vi "Delay Line.vi"() -> ()   [LabVIEW 2013]
uses:
  PI Globals/MercuryConfigured.vi
  PI Globals/ControllerIdentification.vi
  PI Globals/MovementRange.vi
  PI Globals/ConnectedAxes.vi
panel:
  in  "Clear Error":bool
  out "Current velocity":dbl
  in  "Set Velocity":bool
  in  "Set Vel.":dbl
  in  "Query Velocity":bool
  in  "Start":bool
  out "Ready?":bool=TRUE
  in  "JOG +":bool
  out "Conn. \nAxes":string[](array[string])
  in  "Go":bool
  in  "Position to reach":dbl
  in  "Step Size (mm)":dbl
  in  "JOG -":bool
  out "Serial Number":string
  out "Identification":string
  out "+/- Movement range":dbl
  out "error out":errorcluster
  in  "Query Pos.":bool
  out "Position de la ligne à retard":dbl(slide) min=-51.0 max=51.0 scale=0.0..100.0
  in  "error in":errorcluster
  in  "stop":bool
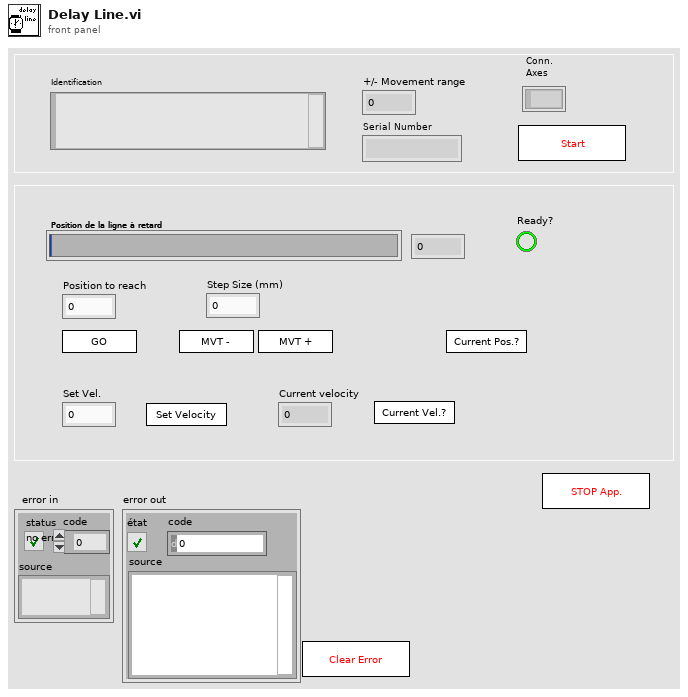
[diagram p1: front panel]
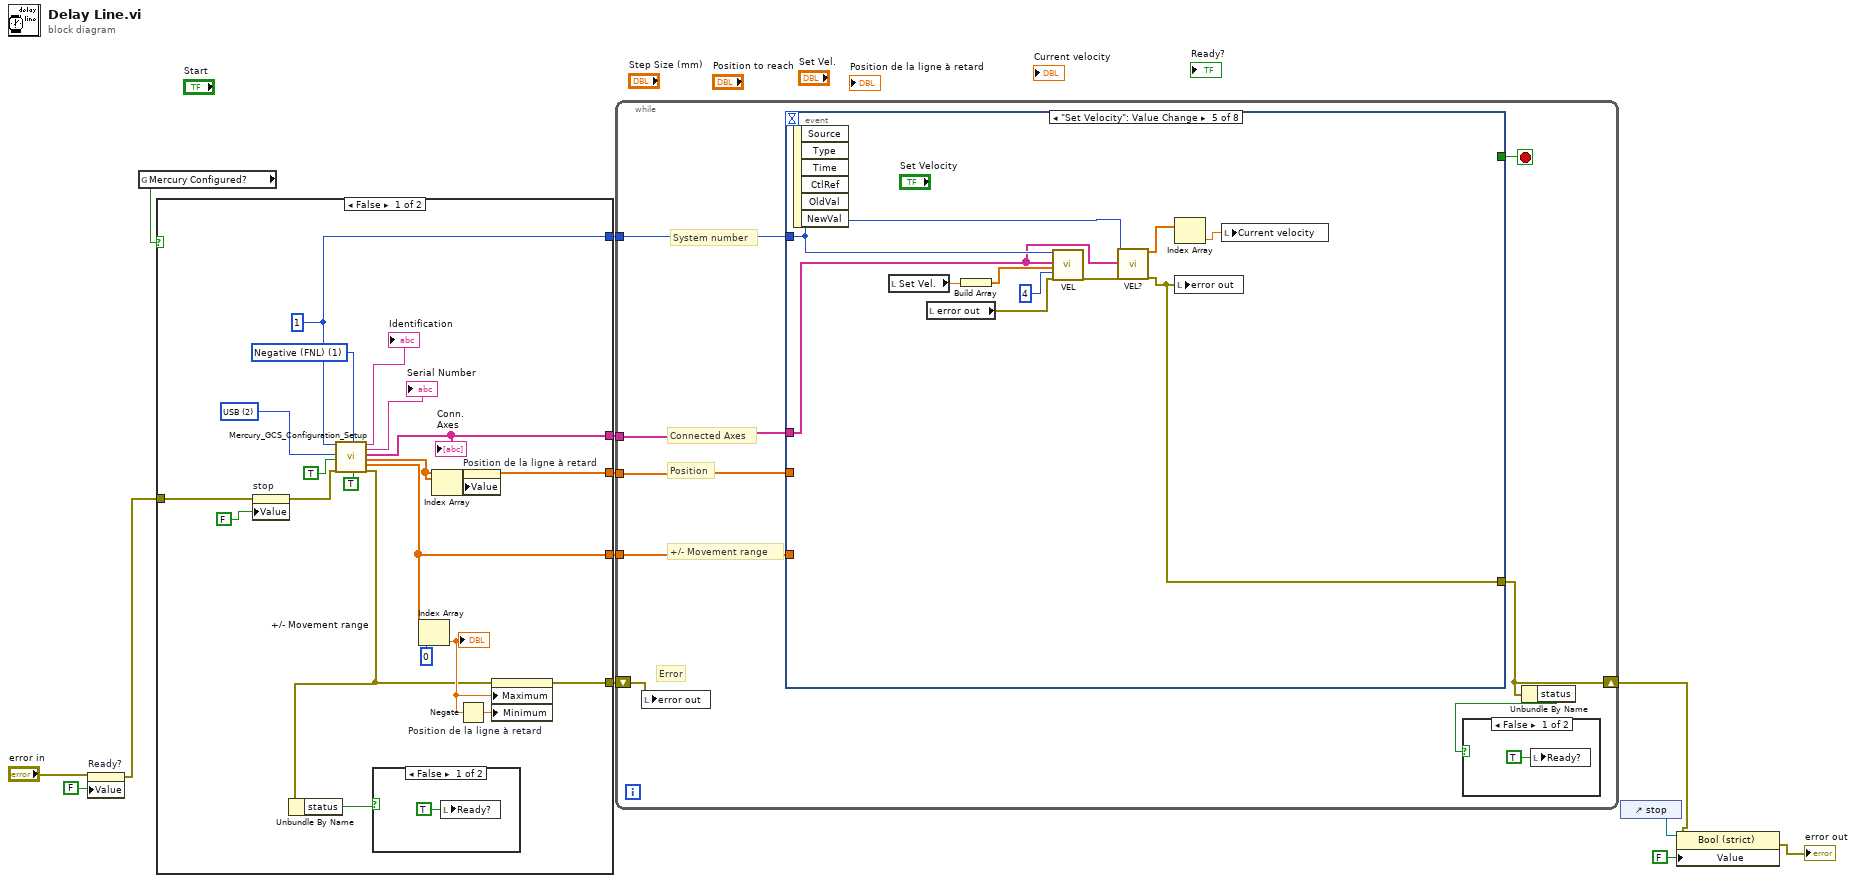
[diagram p0: block diagram]
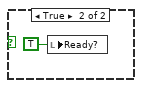
[diagram p2: hidden frame]
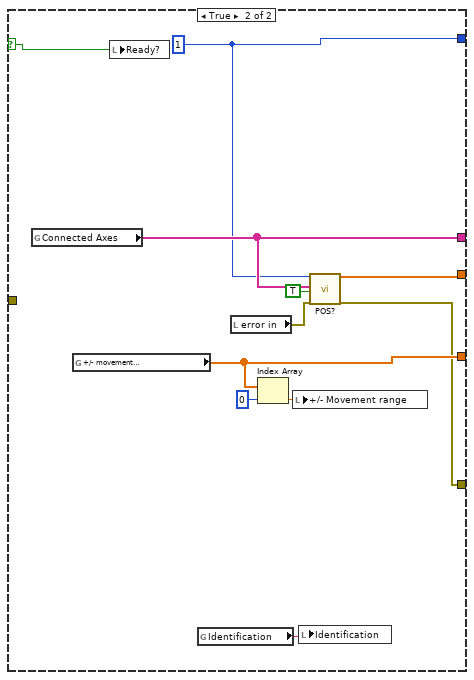
[diagram p3: hidden frame]
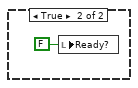
[diagram p4: hidden frame]
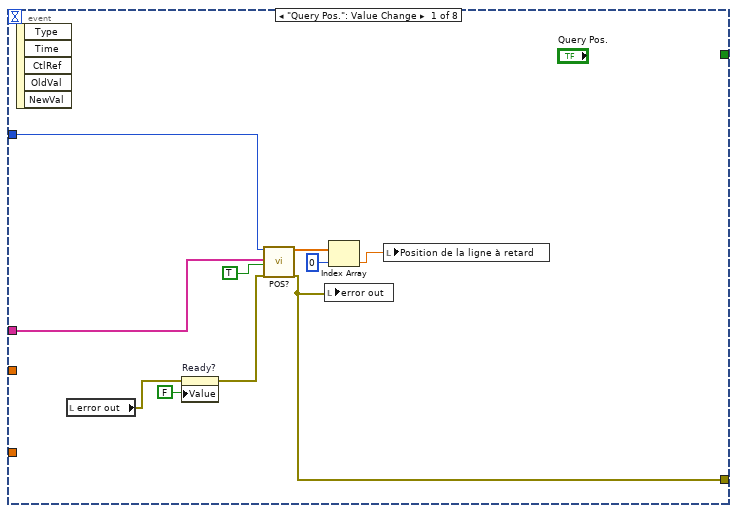
[diagram p5: hidden frame]
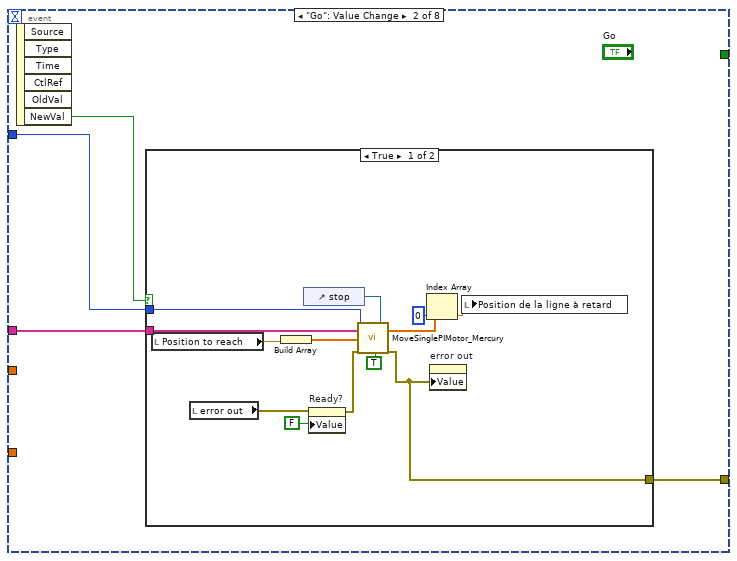
[diagram p6: hidden frame]
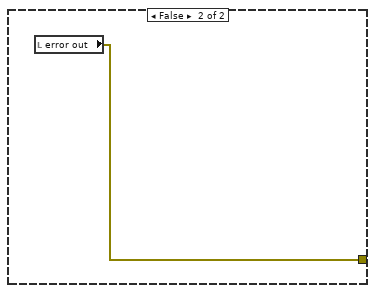
[diagram p7: hidden frame]
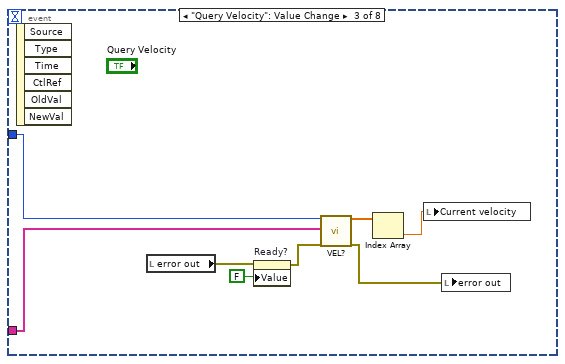
[diagram p8: hidden frame]
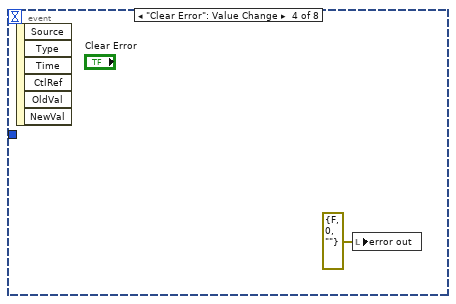
[diagram p9: hidden frame]
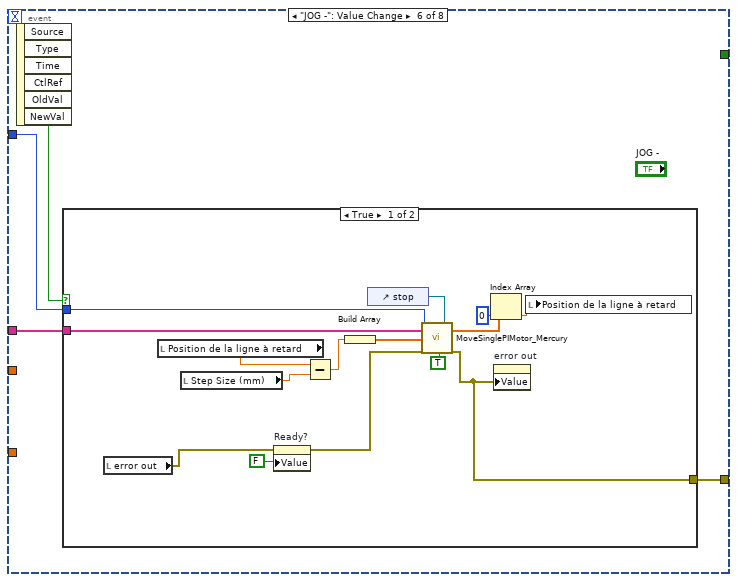
[diagram p10: hidden frame]
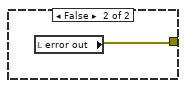
[diagram p11: hidden frame]
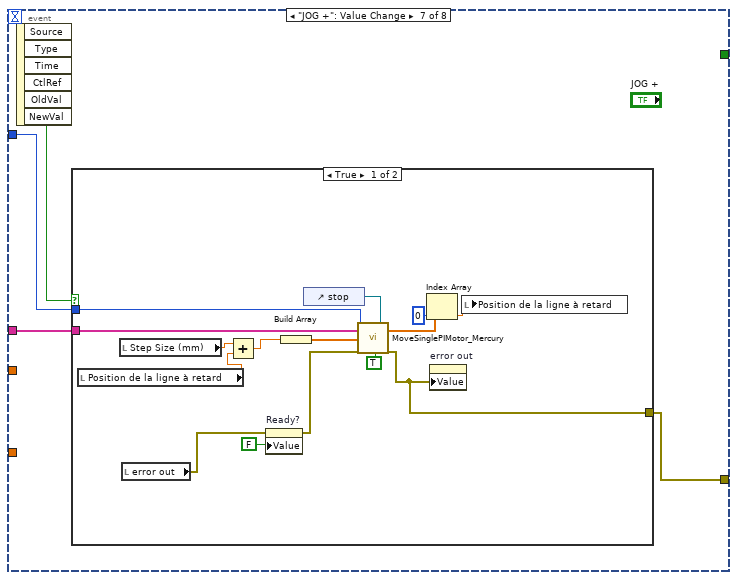
[diagram p12: hidden frame]
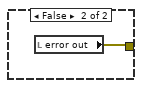
[diagram p13: hidden frame]
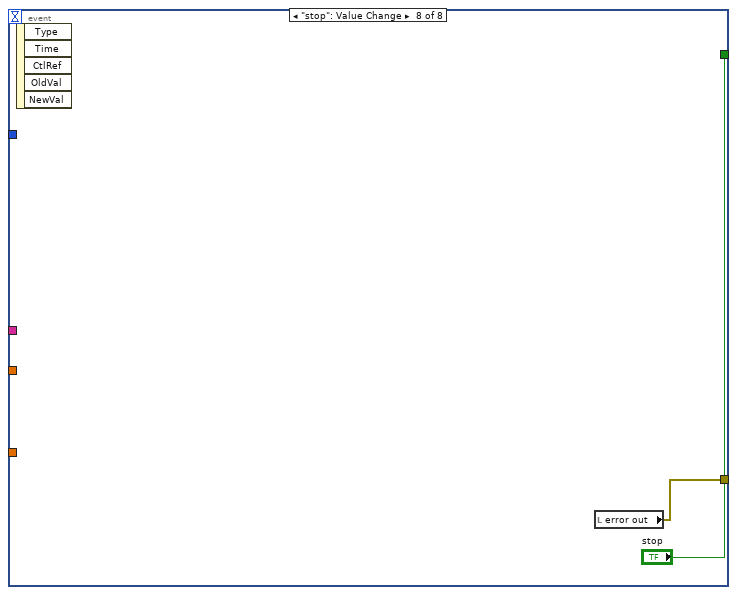
[diagram p14: hidden frame]
diagram:
  n1 = property on="Ready?" class="Bool (strict)"(error in="error in", "Value"=FALSE ("Ready?")) -> (error out=w2:errorcluster)  [unwired: 1 in, 1 out]
  n2 = global read "MercuryConfigured.vi" "Mercury Configured?"() -> (w4:bool)
  n3 = case shown="False" w4 {
    selector: w4 -> [_ w46]
    tunnel: [w31 w40] -> w13
    tunnel: [w26 w39] -> w12
    tunnel: [w24 w43] -> w11
    tunnel: [w23 w37] -> w6
    tunnel: [w16 w45] -> w5
    tunnel: w2 -> [w14 _]
    frame False {
      w32 = u16 1 items=["Positive (FPL)", "Negative (FNL)"] ("Limit switch selection")
      w33 = u16 2 items=["RS232", "RS232 DaisyChain", "USB", "USB_DaisyChain"] ("Interface")
      w26 = 1 ("System no.")
      n4 = property on="stop" class="Bool (strict)"(error in=w14, "Value"=FALSE) -> (error out=w27:errorcluster)  [unwired: 1 in, 1 out]
      n5 = call "Mercury_GCS_Configuration_Setup.vi"("System no."=w26, "Interface"=w33, "All axes?"=TRUE, "error in"=w27, "Reference Move"=w32, "Switch servo on?"=TRUE) -> ("Identification"=→"Identification":string, "SN out"=→"Serial Number":string, "Conn. \nAxes"=w31:string[], "Position"=w16:dbl[], "+/- movement\nrange"=w24:dbl[], "error out"=w18:errorcluster)  [unwired: 7 in, 1 out]
      "Conn. \nAxes" <- w31
      n6 = Unbundle By Name(w18) -> ("status"=w17:bool)
      n7 = case shown="False" w17 {
        frame False {
          n8 = local write "Ready?"(TRUE ("Ready?")) -> ()
        }
        frame True {
          n9 = local write "Ready?"(TRUE ("Ready?")) -> ()
        }
      }
      n10 = Index Array(array=w24, index=0) -> (element=w22:dbl)
      "+/- Movement range" <- w22
      n11 = Index Array(array=w16) -> (element=w15:dbl)  [unwired: 1 in]
      n12 = Negate(x=w22) -> (-x=w21:dbl)
      n13 = property on="Position de la ligne à retard" class="Slide (strict)"("Value"=w15) -> ()  [unwired: 2 in, 2 out]
      n14 = property on="Position de la ligne à retard" class="Slide (strict)"(error in=w18, "Maximum"=w22, "Minimum"=w21) -> (error out=w23:errorcluster)  [unwired: 1 in, 1 out]
    }
    frame True {
      w39 = 1 ("System no.")
      n15 = global read "ConnectedAxes.vi" "Connected Axes"() -> (w40:string[])
      n16 = global read "MovementRange.vi" "+/- movement\nrange"() -> (w43:dbl[])
      n17 = local write "Ready?"(w46) -> ()
      n18 = global read "ControllerIdentification.vi" "Identification"() -> (w44:string)
      n19 = local read "error in"() -> (w36:errorcluster)
      n20 = Index Array(array=w43, index=0 ("indice")) -> (element=w42:dbl)
      n21 = local write "+/- Movement range"(w42) -> ()
      n22 = local write "Identification"(w44) -> ()
      n23 = call "POS?.vi"("System no."=w39, "Axes to query"=w40, "All axes?"=TRUE, "error in"=w36) -> ("Position"=w45:dbl[], "error out"=w37:errorcluster)  [unwired: 14 in]
    }
  }
  n24 = while {
    shift-right: [w48] -> w9
    shift-left: w6 -> [w49]
    tunnel: w13 -> [w54]
    tunnel: w11 -> [w53]
    tunnel: w5 -> [w52]
    tunnel: w12 -> [w51]
    stop <- w50 stop-if-true
    # "System number"
    # "Connected Axes"
    # "Position"
    # "+/- Movement range"
    # "Error"
    n25 = local write "error out"(w49) -> ()
    n26 = event shown="[4] \"Set Velocity\": Value Change" {
      selector: _ -> [_ _ _ _ _ _ _ _]
      dyn-events: _ -> [_ _ _ _ _ _ _ _]
      timeout: _ -> [_ _ _ _ _ _ _ _]
      tunnel: w54 -> [w65 w68 w91 _ w97 w105 w125 _]
      tunnel: w53 -> [_ _ _ _ _ _ _ _]
      tunnel: w52 -> [_ _ _ _ _ _ _ _]
      tunnel: w51 -> [w66 w69 w90 _ w98 w106 w126 _]
      tunnel: [w61 w67 _ _ w94 w104 w124 w144] -> w48
      tunnel: [_ _ _ _ _ _ _ "stop"] -> w50
      event "Query Pos.": Value Change {
        n27 = event-data() -> ()  [unwired: 1 in, 5 out]
        n28 = local read "error out"() -> (w59:errorcluster)
        n29 = property on="Ready?" class="Bool (strict)"(error in=w59, "Value"=FALSE ("Ready?")) -> (error out=w57:errorcluster)  [unwired: 1 in, 1 out]
        n30 = call "POS?.vi"("System no."=w66, "Axes to query"=w65, "All axes?"=TRUE, "error in"=w57) -> ("Position"=w63:dbl[], "error out"=w61:errorcluster)  [unwired: 14 in]
        n31 = local write "error out"(w61) -> ()
        n32 = Index Array(array=w63, index=0) -> (element=w60:dbl)
        n33 = local write "Position de la ligne à retard"(w60) -> ()
      }
      event "Go": Value Change {
        n34 = event-data() -> ("NewVal"=w70:bool)  [unwired: 1 in, 5 out]
        n35 = case shown="True" w70 {
          tunnel: w69 -> [w83 _]
          tunnel: w68 -> [w82 _]
          tunnel: [w76 w84] -> w67
          frame True {
            n36 = local read "Position to reach"() -> (w75:dbl)
            n37 = local read "error out"() -> (w73:errorcluster)
            n38 = Build Array(w75) -> (w74:dbl[])
            n39 = control-ref of="stop"() -> (w80:refnum<vi>)
            n40 = property on="Ready?" class="Bool (strict)"(error in=w73, "Value"=FALSE ("Ready?")) -> (error out=w71:errorcluster)  [unwired: 1 in, 1 out]
            n41 = call "MoveSinglePIMotor_Mercury.vi"("System no."=w83, "Axes to move"=w82, 3:"Move"=w74, "error in"=w71, 11:"Move"=TRUE ("Move"), "Stop refnum"=w80) -> ("Position"=w78:dbl[], "error out"=w76:errorcluster)  [unwired: 12 in]
            n42 = Index Array(array=w78, index=0) -> (element=w77:dbl)
            n43 = property on="error out" class="Clust (strict)"("Value"=w76) -> ()  [unwired: 2 in, 2 out]
            n44 = local write "Position de la ligne à retard"(w77) -> ()
          }
          frame False {
            n45 = local read "error out"() -> (w84:errorcluster)
          }
        }
      }
      event "Query Velocity": Value Change {
        n46 = event-data() -> ()  [unwired: 1 in, 6 out]
        n47 = local read "error out"() -> (w87:errorcluster)
        n48 = property on="Ready?" class="Bool (strict)"(error in=w87, "Value"=FALSE ("Ready?")) -> (error out=w85:errorcluster)  [unwired: 1 in, 1 out]
        n49 = call "VEL?.vi"("System no."=w90, "Axes to query"=w91, "error in"=w85) -> ("Velocity"=w89:dbl[], "error out"=w92:errorcluster)  [unwired: 15 in]
        n50 = Index Array(array=w89) -> (element=w88:dbl)  [unwired: 1 in]
        n51 = local write "Current velocity"(w88) -> ()
        n52 = local write "error out"(w92) -> ()
      }
      event "Clear Error": Value Change {
        n53 = event-data() -> ()  [unwired: 1 in, 6 out]
        n54 = local write "error out"(errorcluster {"status"=FALSE, "code"=0, "source"=""} ("error out")) -> ()
      }
      event "Set Velocity": Value Change {
        n55 = event-data() -> ()  [unwired: 1 in, 6 out]
        n56 = local read "Set Vel."() -> (w101:dbl)
        n57 = local read "error out"() -> (w102:errorcluster)
        n58 = Build Array(w101) -> (w100:dbl[])
        n59 = call "VEL.vi"("System no."=w98, "Axes to set"=w97, "Velocity values"=w100, "No.of digits"=i16 4, "error in"=w102) -> ("error out"=w99:errorcluster)  [unwired: 13 in, 1 out]
        n60 = call "VEL?.vi"("System no."=w98, "Axes to query"=w97, "error in"=w99) -> ("Velocity"=w96:dbl[], "error out"=w94:errorcluster)  [unwired: 15 in]
        n61 = Index Array(array=w96) -> (element=w95:dbl)  [unwired: 1 in]
        n62 = local write "error out"(w94) -> ()
        n63 = local write "Current velocity"(w95) -> ()
      }
      event "JOG -": Value Change {
        n64 = event-data() -> ("NewVal"=w107:bool)  [unwired: 1 in, 5 out]
        n65 = case shown="True" w107 {
          tunnel: w106 -> [w122 _]
          tunnel: w105 -> [w121 _]
          tunnel: [w115 w123] -> w104
          frame True {
            n66 = local read "error out"() -> (w110:errorcluster)
            n67 = local read "Position de la ligne à retard"() -> (w113:dbl)
            n68 = local read "Step Size (mm)"() -> (w112:dbl)
            n69 = property on="Ready?" class="Bool (strict)"(error in=w110, "Value"=FALSE ("Ready?")) -> (error out=w108:errorcluster)  [unwired: 1 in, 1 out]
            n70 = Subtract(x=w113, y=w112) -> (x-y=w114:dbl)
            n71 = Build Array(w114) -> (w111:dbl[])
            n72 = control-ref of="stop"() -> (w119:refnum<vi>)
            n73 = call "MoveSinglePIMotor_Mercury.vi"("System no."=w122, "Axes to move"=w121, 3:"Move"=w111, "error in"=w108, 11:"Move"=TRUE ("Move"), "Stop refnum"=w119) -> ("Position"=w117:dbl[], "error out"=w115:errorcluster)  [unwired: 12 in]
            n74 = Index Array(array=w117, index=0) -> (element=w116:dbl)
            n75 = property on="error out" class="Clust (strict)"("Value"=w115) -> ()  [unwired: 2 in, 2 out]
            n76 = local write "Position de la ligne à retard"(w116) -> ()
          }
          frame False {
            n77 = local read "error out"() -> (w123:errorcluster)
          }
        }
      }
      event "JOG +": Value Change {
        n78 = event-data() -> ("NewVal"=w127:bool)  [unwired: 1 in, 5 out]
        n79 = case shown="True" w127 {
          tunnel: w126 -> [w142 _]
          tunnel: w125 -> [w141 _]
          tunnel: [w131 w143] -> w124
          frame True {
            n80 = local read "Position de la ligne à retard"() -> (w134:dbl)
            n81 = local read "Step Size (mm)"() -> (w135:dbl)
            n82 = local read "error out"() -> (w129:errorcluster)
            n83 = Add(x=w135, y=w134) -> (x+y=w133:dbl)
            n84 = property on="Ready?" class="Bool (strict)"(error in=w129, "Value"=FALSE ("Ready?")) -> (error out=w128:errorcluster)  [unwired: 1 in, 1 out]
            n85 = Build Array(w133) -> (w132:dbl[])
            n86 = control-ref of="stop"() -> (w139:refnum<vi>)
            n87 = call "MoveSinglePIMotor_Mercury.vi"("System no."=w142, "Axes to move"=w141, 3:"Move"=w132, "error in"=w128, 11:"Move"=TRUE ("Move"), "Stop refnum"=w139) -> ("Position"=w137:dbl[], "error out"=w131:errorcluster)  [unwired: 12 in]
            n88 = Index Array(array=w137, index=0) -> (element=w136:dbl)
            n89 = property on="error out" class="Clust (strict)"("Value"=w131) -> ()  [unwired: 2 in, 2 out]
            n90 = local write "Position de la ligne à retard"(w136) -> ()
          }
          frame False {
            n91 = local read "error out"() -> (w143:errorcluster)
          }
        }
      }
      event "stop": Value Change {
        n92 = event-data() -> ()  [unwired: 1 in, 5 out]
        n93 = local read "error out"() -> (w144:errorcluster)
      }
    }
    n94 = Unbundle By Name(w48) -> ("status"=w47:bool)
    n95 = case shown="False" w47 {
      frame False {
        n96 = local write "Ready?"(TRUE ("Ready?")) -> ()
      }
      frame True {
        n97 = local write "Ready?"(FALSE ("Ready?")) -> ()
      }
    }
  }
  n98 = control-ref of="stop"() -> (w10:refnum<vi>)
  n99 = property class="Bool (strict)"(reference=w10, error in=w9, "Value"=FALSE) -> (error out=→"error out":errorcluster)  [unwired: 1 out]
